vi "From URL.vi"(8 "error in (no error)":errorcluster, 10 "Feed URL":string) -> (0 "error out":errorcluster, 1 "feed valid?":bool, 2 "url valid?":bool, 3 "Feed out":refnum<class "Feed.lvclass">)   [LabVIEW 2020, in "Feed.lvclass"]
uses:
  <vilib>/NI_RSS/Feed/Feed.lvclass
  <vilib>/NI_RSS/FeedItem/FeedItem.lvclass
  <vilib>/NI_RSS/Feed/Feed.lvclass/Feed.ctl
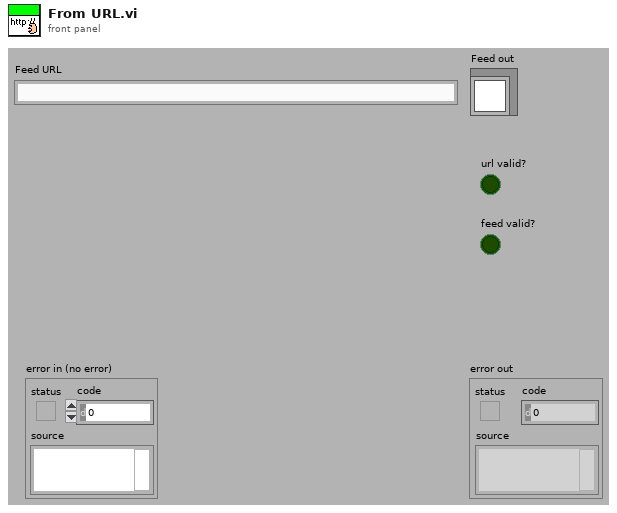
[diagram p1: front panel]
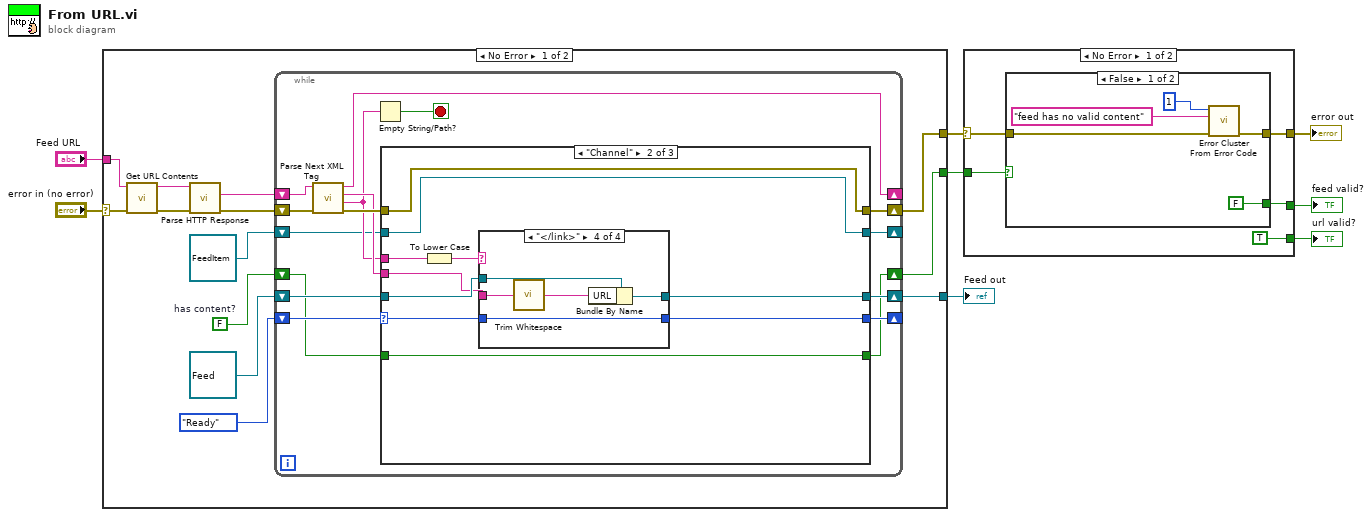
[diagram p0: block diagram]
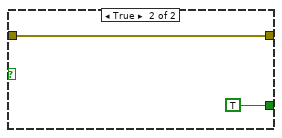
[diagram p2: hidden frame]
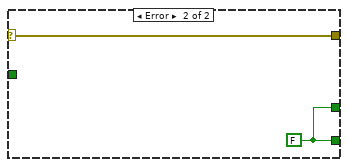
[diagram p3: hidden frame]
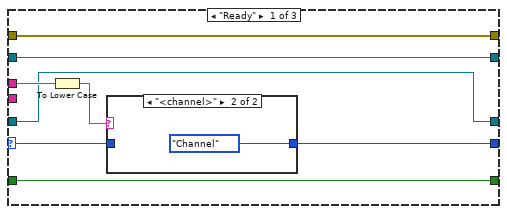
[diagram p4: hidden frame]
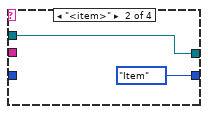
[diagram p7: hidden frame]
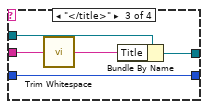
[diagram p8: hidden frame]
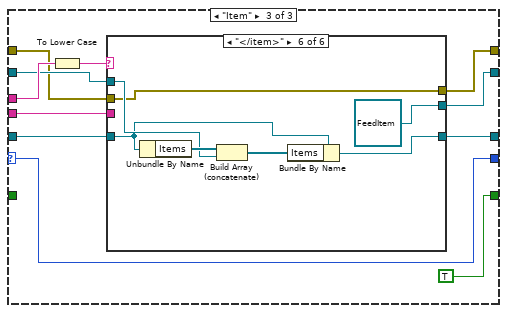
[diagram p9: hidden frame]
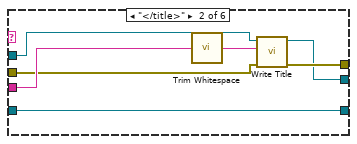
[diagram p11: hidden frame]
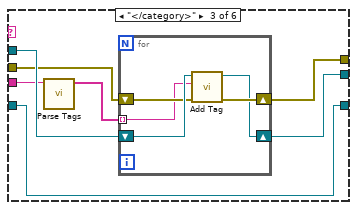
[diagram p12: hidden frame]
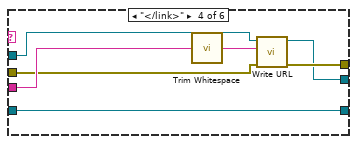
[diagram p13: hidden frame]
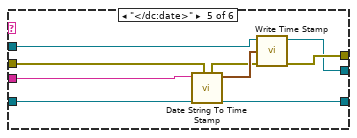
[diagram p14: hidden frame]
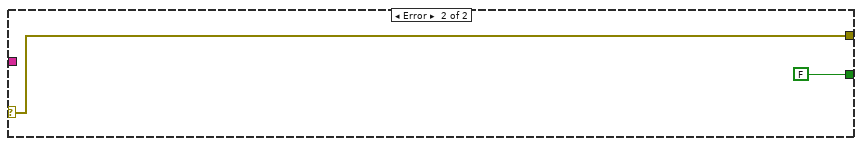
[diagram p15: hidden frame]
diagram:
  n1 = case shown="No Error" "error in (no error)" {
    selector: "error in (no error)" -> [w20 w128]
    tunnel: [w12 w128] -> w5
    tunnel: [w13 _] -> w7
    tunnel: "Feed URL" -> [w19 _]
    tunnel: [w9 FALSE ("has content?")] -> w4
    frame No Error {
      w10 = FALSE  # has content?
      n2 = call <vilib>:"Get URL Contents.vi"("error in (no error)"=w20, "URL"=w19) -> ("error out"=w21:errorcluster, "Contents"=w18:string)  [unwired: 1 in, 7 out]
      n3 = call <vilib>:"Parse HTTP Response.vi"("error in (no error)"=w21, "HTTP Response"=w18) -> ("error out"=w17:errorcluster, "Body"=w16:string)  [unwired: 8 out]
      n4 = while {
        shift-right: [w35] -> _
        shift-left: w16 -> [w37]
        shift-right: [w31] -> _
        shift-left: enum16{"Ready", "Channel", "Item"}."Ready" -> [w34]
        shift-right: [w29] -> w13
        shift-left: refnum<class "Feed.lvclass"> refnum ("Feed out") -> [w30]
        shift-right: [w26] -> w12
        shift-left: w17 -> [w36]
        shift-right: [w24] -> _
        shift-left: refnum<class "FeedItem.lvclass"> refnum ("FeedItem.lvclass") -> [w25]
        shift-right: [w22] -> w9
        shift-left: w10 -> [w23]
        stop <- w27 stop-if-true
        n5 = call <vilib>:"Parse Next XML Tag.vi"("error in (no error)"=w36, "XML in"=w37) -> ("error out"=w33:errorcluster, "Tag"=w28:string, "Before Tag"=w32:string, "XML out"=w35:string)  [unwired: 6 out]
        n6 = Empty String/Path?(string/path=w28) -> (empty?=w27:bool)
        n7 = case shown="\"Channel\"" w34 {
          selector: w34 -> [w42 w51 w80]
          tunnel: w28 -> [w45 w57 w81]
          tunnel: w33 -> [w40 w50 w77]
          tunnel: w32 -> [_ w53 w78]
          tunnel: [w43 w52 w80] -> w31
          tunnel: w30 -> [w41 w55 w74]
          tunnel: [w41 w54 w73] -> w29
          tunnel: [w40 w50 w76] -> w26
          tunnel: w25 -> [w39 w49 w79]
          tunnel: [w39 w49 w75] -> w24
          tunnel: w23 -> [w38 w48 _]
          tunnel: [w38 w48 TRUE ("has content?")] -> w22
          frame "Ready" {
            n8 = To Lower Case(string=w45) -> (all lower case string=w44:string)
            n9 = case shown="\"<channel>\"" w44 {
              tunnel: [w46 enum16{"Ready", "Channel", "Item"}."Channel"] -> w43
              tunnel: w42 -> [w46 _]
              frame Default {
              }
              frame "<channel>" {
              }
            }
          }
          frame "Channel" {
            n10 = To Lower Case(string=w57) -> (all lower case string=w56:string)
            n11 = case shown="\"</link>\"" w56 {
              tunnel: w55 -> [w59 w61 w64 w69]
              tunnel: [w59 w61 w63 w68] -> w54
              tunnel: w53 -> [_ _ w66 w71]
              tunnel: [w58 enum16{"Ready", "Channel", "Item"}."Item" w62 w67] -> w52
              tunnel: w51 -> [w58 _ w62 w67]
              frame Default {
              }
              frame "<item>" {
              }
              frame "</title>" {
                n12 = call <vilib>:"Trim Whitespace.vi"("string"=w66) -> ("trimmed string"=w65:string)  [unwired: 1 in]
                n13 = Bundle By Name(cluster=w64, "Title"=w65) -> (w63:refnum<class "Feed.lvclass">)
              }
              frame "</link>" {
                n14 = call <vilib>:"Trim Whitespace.vi"("string"=w71) -> ("trimmed string"=w70:string)  [unwired: 1 in]
                n15 = Bundle By Name(cluster=w69, "URL"=w70) -> (w68:refnum<class "Feed.lvclass">)
              }
            }
          }
          frame "Item" {
            n16 = To Lower Case(string=w81) -> (all lower case string=w82:string)
            n17 = case shown="\"</item>\"" w82 {
              tunnel: w79 -> [w84 w92 w99 w111 w119 w125]
              tunnel: w78 -> [_ w91 w94 w110 w115 _]
              tunnel: w77 -> [w85 w89 w98 w108 w113 w120]
              tunnel: [w85 w88 w97 w107 w118 w120] -> w76
              tunnel: [w84 w87 w96 w106 w117 refnum<class "FeedItem.lvclass"> refnum ("FeedItem.lvclass out")] -> w75
              tunnel: w74 -> [w83 w86 w95 w105 w116 w124]
              tunnel: [w83 w86 w95 w105 w116 w122] -> w73
              frame Default {
              }
              frame "</title>" {
                n18 = call <vilib>:"Trim Whitespace.vi"("string"=w91) -> ("trimmed string"=w90:string)  [unwired: 1 in]
                n19 = call-dynamic "Write Title.vi"("error in (no error)"=w89, "Title"=w90, "FeedItem.lvclass in"=w92) -> ("error out"=w88:errorcluster, "FeedItem.lvclass out"=w87:refnum<class "FeedItem.lvclass">)  [unwired: 7 out]
              }
              frame "</category>" {
                n20 = call <vilib>:"Parse Tags.vi"("Tags"=w94) -> ("Tags"=w93:string[])  [unwired: 10 out]
                n21 = for {
                  shift-right: [w101] -> w96
                  shift-left: w99 -> [w104]
                  shift-right: [w102] -> w97
                  shift-left: w98 -> [w103]
                  tunnel: w93 -> [w100] mode=indexing
                  n22 = call-dynamic "Add Tag.vi"("error in (no error)"=w103, "Tag"=w100, "FeedItem.lvclass in"=w104) -> ("error out"=w102:errorcluster, "FeedItem.lvclass out"=w101:refnum<class "FeedItem.lvclass">)  [unwired: 7 out]
                }
              }
              frame "</link>" {
                n23 = call <vilib>:"Trim Whitespace.vi"("string"=w110) -> ("trimmed string"=w109:string)  [unwired: 1 in]
                n24 = call-dynamic "Write URL.vi"("error in (no error)"=w108, "URL"=w109, "FeedItem.lvclass in"=w111) -> ("error out"=w107:errorcluster, "FeedItem.lvclass out"=w106:refnum<class "FeedItem.lvclass">)  [unwired: 7 out]
              }
              frame "</dc:date>" {
                n25 = call <vilib>:"Date String To Time Stamp.vi"("error in (no error)"=w113, "Date"=w115) -> ("Time Stamp"=w114:timestamp, "error out"=w112:errorcluster)  [unwired: 8 out]
                n26 = call-dynamic "Write Time Stamp.vi"("error in (no error)"=w112, "Time Stamp"=w114, "FeedItem.lvclass in"=w119) -> ("error out"=w118:errorcluster, "FeedItem.lvclass out"=w117:refnum<class "FeedItem.lvclass">)  [unwired: 7 out]
              }
              frame "</item>" {
                n27 = Unbundle By Name(w124) -> ("Items"=w126:refnum<class "FeedItem.lvclass">[])
                n28 = Build Array (concatenate)(w126, w125) -> (w123:refnum<class "FeedItem.lvclass">[])
                n29 = Bundle By Name(cluster=w124, "Items"=w123) -> (w122:refnum<class "Feed.lvclass">)
              }
            }
          }
        }
      }
    }
    frame Error {
    }
  }
  "Feed out" <- w7
  n30 = case shown="No Error" w5 {
    selector: w5 -> [w132 w142]
    tunnel: w4 -> [w133 _]
    tunnel: [w131 w142] -> w3
    tunnel: [TRUE w141] -> w2
    tunnel: [w129 w141] -> w1
    frame No Error {
      n31 = case shown="False" w133 {
        tunnel: [w135 w140] -> w131
        tunnel: w132 -> [w136 w140]
        tunnel: [FALSE TRUE] -> w129
        frame False {
          n32 = call <vilib>:"Error Cluster From Error Code.vi"("error in (no error)"=w136, "error message (\"\")"="feed has no valid content" ("source"), "error code (0)"=1 ("code")) -> ("error out"=w135:errorcluster)  [unwired: 1 in, 5 out]
        }
        frame True {
        }
      }
    }
    frame Error {
      w141 = FALSE
    }
  }
  "error out" <- w3
  "url valid?" <- w2
  "feed valid?" <- w1
